vi "Resolve Local Data.vi"(6 "Promise":refnum<class "Promise.lvclass">, 8 "error in (no error)":errorcluster, 10 "Data Request":T1, 11 "Historian Module in":refnum<class "Historian Module.lvclass">) -> (0 "error out":errorcluster, 3 "Historian Module out":refnum<class "Historian Module.lvclass">)   [LabVIEW 2020, in "VolatusHistorian.lvlib" / "Historian Module.lvclass"]
uses:
  Historian Module.lvclass
  Historian Module.lvclass/Historian Module.ctl
  History Data Value/Unix ns Data Value.lvclass
  Local Data Value/LV Dbl Data Value.lvclass
  lv-promises/Promises/Promise/Promise.lvclass
  C:/dev/lv20CE/relink/lv-promises/Promises/Value/Value.lvclass
  C:/dev/lv20CE/relink/lv-volatus/VolatusHistorian/History Data Value/Unix ns Data Value.lvclass
  C:/dev/lv20CE/relink/lv-volatus/VolatusHistorian/Local Data Value/LV Dbl Data Value.lvclass
  Time Format.ctl
  VolatusHistorian.lvlib
  Data Request.ctl
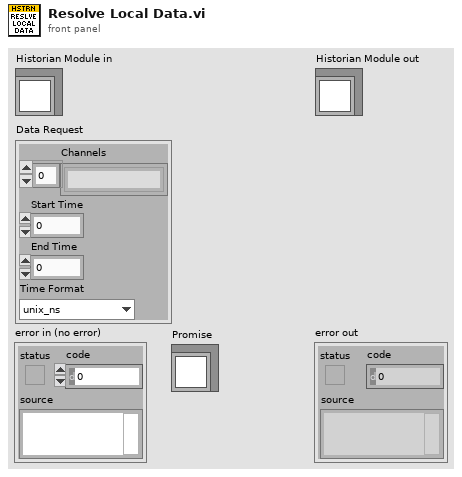
[diagram p1: front panel]
types:
  T1 = typedef "VolatusHistorian.lvlib/Data Request.ctl" = cluster{"Channels":string[], "Start Time":dbl, "End Time":dbl, "Time Format":T2}
  T2 = typedef "VolatusHistorian.lvlib/Time Format.ctl" = enum16{"unix_ns", "lv"}
  T3 = typedef "VolatusHistorian.lvlib/History Data (unix ns).ctl" = cluster{"Channels":T4[]}
  T4 = typedef "VolatusHistorian.lvlib/Channel History (unix ns).ctl" = cluster{"Name":string, "Unix_ns":i64[], "Data":dbl[]}
  T5 = typedef "VolatusHistorian.lvlib/History Data (LV Dbl).ctl" = cluster{"Channels":T6[]}
  T6 = typedef "VolatusHistorian.lvlib/Channel History (LV Dbl).ctl" = cluster{"Name":string, "Timestamps":dbl[], "Data":dbl[]}
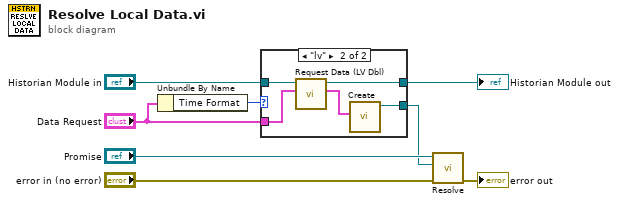
[diagram p0: block diagram]
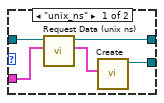
[diagram p2: hidden frame]
diagram:
  n1 = Unbundle By Name("Data Request") -> ("Time Format"=w7:T2)
  n2 = case shown="\"lv\"" w7 {
    tunnel: "Historian Module in" -> [w13 w18]
    tunnel: "Data Request" -> [w12 w17]
    tunnel: [w10 w16] -> w5
    tunnel: [w9 w14] -> w3
    frame "unix_ns" {
      n3 = call "Request Data (unix ns).vi"("Data Request"=w12, "Historian Module in"=w13) -> ("History Data"=w11:T3, "Historian Module out"=w10:refnum<class "Historian Module.lvclass">)  [unwired: 8 in]
      n4 = call "Create.vi"("Data"=w11) -> ("History Data Value out"=w9:refnum<class "Unix ns Data Value.lvclass">)  [unwired: 10 in]
    }
    frame "lv" {
      n5 = call "Request Data (LV Dbl).vi"("Data Request"=w17, "Historian Module in"=w18) -> ("Local History"=w15:T5, "Historian Module out"=w16:refnum<class "Historian Module.lvclass">)  [unwired: 8 in]
      n6 = call "Create.vi"("Data"=w15) -> ("Local Data Value out"=w14:refnum<class "LV Dbl Data Value.lvclass">)  [unwired: 10 in]
    }
  }
  "Historian Module out" <- w5
  n7 = call "Resolve.vi"("error in (no error)"="error in (no error)", "Result"=w3, "Promise in"="Promise") -> ("error out"=→"error out":errorcluster)  [unwired: 7 in, 1 out]
